vi "Config_Image_Read_CornerROIs.vi"(8 "error in (no error)":errorcluster) -> (0 "error out":errorcluster)   [LabVIEW 2020]
uses:
  <vilib>/Utility/config.llb/Read Key (String).vi
  <vilib>/Utility/config.llb/NI_LVConfig.lvlib
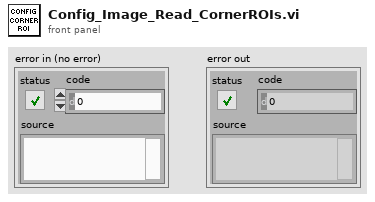
[diagram p1: front panel]
types:
  T1 = typedef "Image_Cluster.ctl" = cluster{"Detector_info":cluster{"No. of detectors":dbl, "Detector_Array":string[][], "Detector_Array_Numeric":dbl[][]}, "Corner_info":cluster{"Corner_Array":dbl[][]}, "ROI":cluster{"Corners":cluster{"Global Rectangle":i32[], "Contours":cluster{"ID":enum32{"External", "Internal"}, "Type":u32, "Coordinates":i32[]}[]}[], "Detectors":cluster{"Global Rectangle":i32[], "Contours":cluster{"ID":enum32{"External", "Internal"}, "Type":u32, "Coordinates":i32[]}[]}[]}, "Shape_Detect":cluster{"Match_score":dbl, "Curve Parameters":T2, "Match Options":T3, "Circle Descriptor":cluster{"Min Radius":dbl, "Max Radius":dbl}}, "Path":cluster{"Config":path, "Map":path}, "Map":cluster{"X":i32, "Y":i32}}
  T2 = typedef "IMAQ Curve Parameters.ctl" = cluster{"Extraction Mode":u32, "Edge Threshold":i32, "Edge Filter Size":u32, "Min Length":i32, "Row Search Step Size":i32, "Col Search Step Size":i32, "Max Endpoint Gap":i32, "Closed":bool, "Subpixel":bool}
  T3 = typedef "ShapeDetectionMatchOptions.ctl" = cluster{"Rotation":bool, "Scale":bool, "Occlusion":bool, "Range Settings":T4[]}
  T4 = typedef "IMAQ Match Range Setting.ctl" = cluster{"Match Constraints":u32, "Min":dbl, "Max":dbl}
  T5 = typedef "NI_LVConfig.lvlib/Config Data RefNum.ctl" = refnum<k1>
  T6 = cluster{"Global Rectangle":i32[], "Contours":cluster{"ID":enum32{"External", "Internal"}, "Type":u32, "Coordinates":i32[]}[]}
  T7 = cluster{"Global Rectangle":i32[], "Contours":cluster{"ID":enum32{"External", "Internal"}, "Type":u32, "Coordinates":i32[]}[]}[]
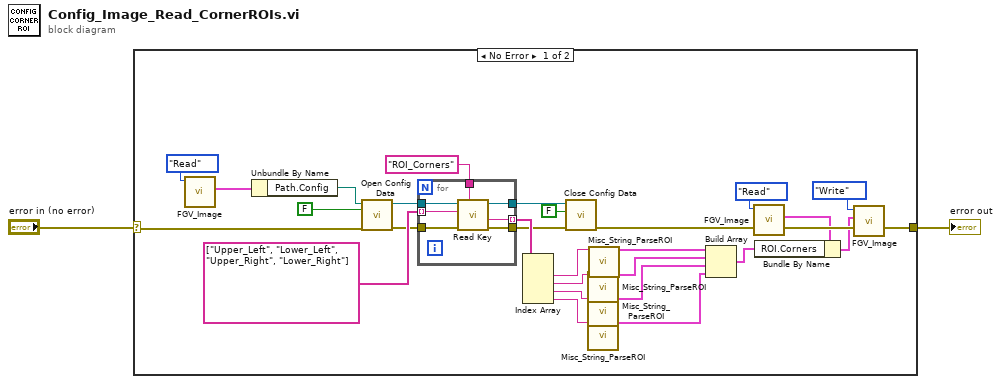
[diagram p0: block diagram]
diagram:
  n1 = case shown="No Error" "error in (no error)" {
    selector: "error in (no error)" -> [w3 w37]
    tunnel: [w29 w37] -> w2
    frame No Error {
      n2 = call "FGV_Image.vi"("Action"=enum16{"Read", "Write", ""}."Read") -> ("Image_Cluster_out"=w27:T1)  [unwired: 10 in]
      n3 = Unbundle By Name(w27) -> ("Path.Config"=w28:path)
      n4 = call <vilib>:"Open Config Data.vi"("error in (no error)"=w3, "create file if necessary (T)"=FALSE, "configuration file path"=w28) -> ("error out"=w9:errorcluster, "refnum"=w8:T5)  [unwired: 6 in, 1 out]
      n5 = for {
        tunnel: w8 -> [w36]
        tunnel: w9 -> [w35]
        tunnel: [w34] -> w6
        tunnel: string[] ["Upper_Left", "Lower_Left", "Upper_Right", "Lower_Right"] ("key names") -> [w33] mode=indexing
        tunnel: "ROI_Corners" -> [w32]
        tunnel: [w30] -> w11 mode=indexing
        tunnel: [w31] -> w7
        n6 = call-poly <vilib>:"Read Key.vi"("section"=w32, "error in (no error)"=w35, "key"=w33, "refnum"=w36) -> ("error out"=w34:errorcluster, "value"=w30:string, "refnum out"=w31:T5)  [unwired: 4 in, 1 out]
      }
      n7 = Index Array(array=w11) -> (element #1=w13:string, element #2=w14:string, element #3=w15:string, element #4=w16:string)  [unwired: 4 in]
      n8 = call <vilib>:"Close Config Data.vi"("error in (no error)"=w6, "write file if changed (T)"=FALSE ("write configuration file? (T)"), "refnum"=w7) -> ("error out"=w29:errorcluster)  [unwired: 8 out]
      n9 = call "Misc_String_ParseROI.vi"("ROI_string"=w14) -> ("ROI"=w20:T6)  [unwired: 14 in]
      n10 = call "Misc_String_ParseROI.vi"("ROI_string"=w15) -> ("ROI"=w21:T6)  [unwired: 14 in]
      n11 = call "Misc_String_ParseROI.vi"("ROI_string"=w16) -> ("ROI"=w22:T6)  [unwired: 14 in]
      n12 = call "Misc_String_ParseROI.vi"("ROI_string"=w13) -> ("ROI"=w19:T6)  [unwired: 14 in]
      n13 = Build Array(w19, w20, w21, w22) -> (w23:T7)
      n14 = call "FGV_Image.vi"("Action"=enum16{"Read", "Write", ""}."Read") -> ("Image_Cluster_out"=w18:T1)  [unwired: 10 in]
      n15 = Bundle By Name(cluster=w18, "ROI.Corners"=w23) -> (w24:T1)
      n16 = call "FGV_Image.vi"("Image_Cluster_in"=w24, "Action"=enum16{"Read", "Write", ""}."Write") -> ()  [unwired: 9 in, 1 out]
    }
    frame Error {
    }
  }
  "error out" <- w2
